vi "波形函数选板讲解.vi"() -> ()   [LabVIEW 2018]
uses:
  <vilib>/Waveform/WDTOps.llb/WDT Append Waveforms DBL.vi
  <vilib>/Waveform/WDTOps.llb/WDT Waveform to XY Pairs DBL.vi
  <vilib>/Waveform/WDTOps.llb/WDT Waveform Duration DBL.vi
panel:
  out "XY图":cluster{"x":timestamp, "y":dbl}[](graph)
  out "波形图 4":waveform(dbl)(graph)
  out "offset":dbl caption="偏移量" format="%0.2f"
  out "scale":dbl caption="比例因子" format="%0.2f"
  out "波形图 3":waveform(dbl)(graph)
  out "波形图 2":waveform(dbl)(graph)
  out "Y":dbl[](array[numeric])
  out "dt":dbl
  out "t0":timestamp
  out "duration":dbl caption="持续时间" format="%0.2f"
  out "波形图":waveform(dbl)(graph)
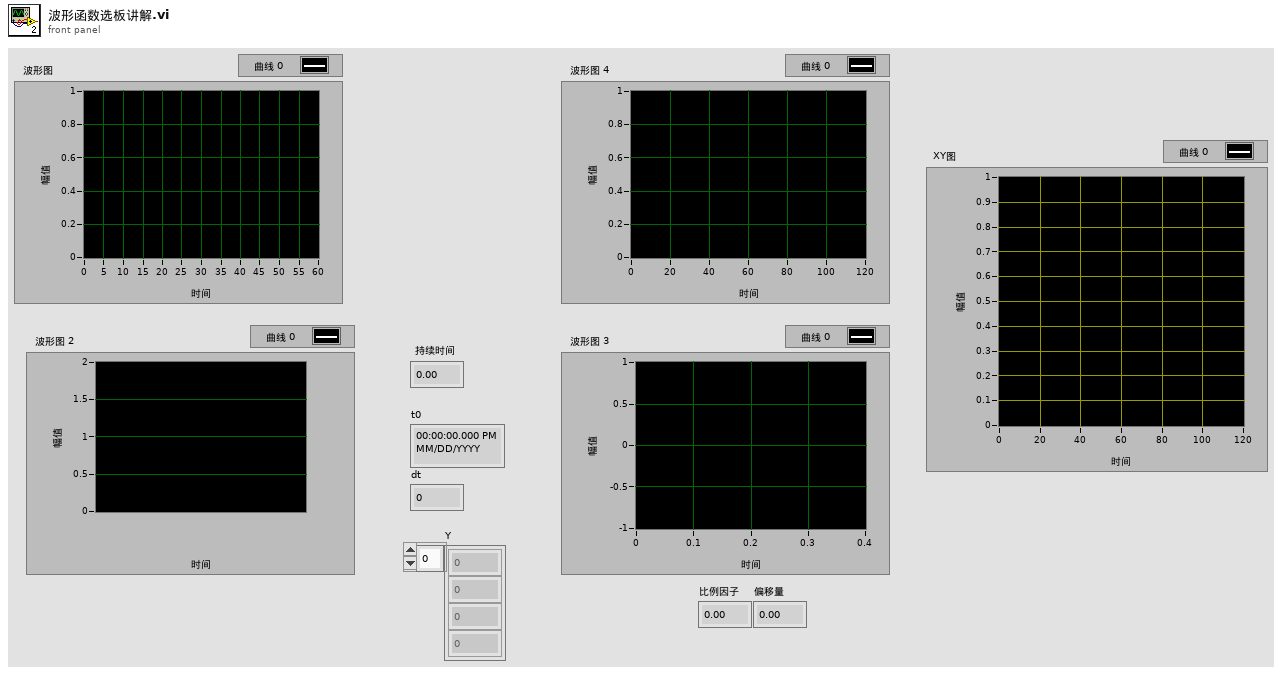
[diagram p1: front panel]
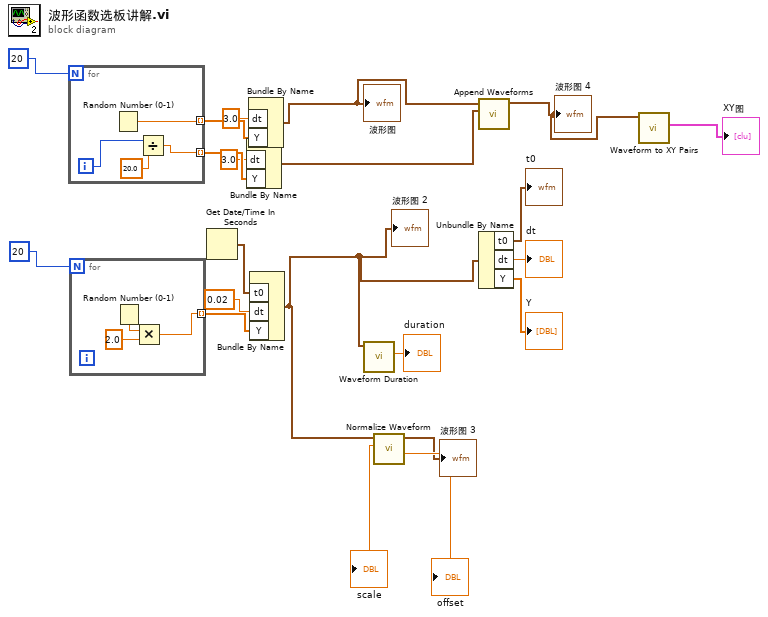
[diagram p0: block diagram]
diagram:
  n1 = for {
    N: 20 -> [_]
    tunnel: [w25] -> w20 mode=indexing
    tunnel: [w22] -> w9 mode=indexing
    i -> [w24]
    n2 = Random Number (0-1)() -> (number: 0 to 1=w25:dbl)
    n3 = Divide(x=w24, y=20.0) -> (x/y=w22:dbl)
  }
  n4 = for {
    N: 20 -> [_]
    tunnel: [w26] -> w18 mode=indexing
    n5 = Random Number (0-1)() -> (number: 0 to 1=w27:dbl)
    n6 = Multiply(x=w27, y=2.0) -> (x*y=w26:dbl)
  }
  n7 = Get Date/Time In Seconds() -> (seconds since 1Jan1904=w17:timestamp)
  n8 = Bundle By Name("dt"=3.0, "Y"=w9) -> (w7:waveform(dbl))  [unwired: 1 in]
  n9 = Bundle By Name("dt"=3.0, "Y"=w20) -> (w8:waveform(dbl))  [unwired: 1 in]
  "波形图" <- w8
  n10 = Bundle By Name("t0"=w17, "dt"=0.02, "Y"=w18) -> (w2:waveform(dbl))  [unwired: 1 in]
  "波形图 2" <- w2
  n11 = call-poly <vilib>:"Waveform Duration.vi"("waveform in"=w2) -> ("duration"=→"duration":dbl)  [unwired: 8 in, 2 out]
  n12 = call <vilib>:"Normalize Waveform.vi"("waveform in"=w2) -> ("offset"=→"offset":dbl, "scale"=→"scale":dbl, "normalized waveform"=→"波形图 3":waveform(dbl))  [unwired: 7 in, 1 out]
  n13 = call-poly <vilib>:"Append Waveforms.vi"("waveform B"=w7, "waveform A"=w8) -> ("waveform out"=w1:waveform(dbl))  [unwired: 8 in, 1 out]
  "波形图 4" <- w1
  n14 = Unbundle By Name(w2) -> ("t0"=→"t0":timestamp, "dt"=→"dt":dbl, "Y"=→"Y":dbl[])
  n15 = call-poly <vilib>:"Waveform to XY Pairs.vi"("waveform in"=w1) -> ("XY pairs"=→"XY图":cluster{"x":timestamp, "y":dbl}[])  [unwired: 8 in, 2 out]
